vi "Configure Trigger (USB).vi"(0 "VISA resource name":refnum<visa-resource-name>, 1 "Split Transaction Start/End (0: No Care)":u16(ring) items=["No Care", "Full Speed", "Low Speed", "ISO Start", "ISO Middle", "ISO End", "ISO All"], 2 "Split Transaction Field (0: No Care)":u16(ring) items=["No Care", "S Split", "C Split"], 5 "Trigger Source (9: Bus 1)":u16(ring)=9 items=["Bus 1"=9, "Bus 2"=10], 7 "Split Transaction Hub Address (\"XXXXXXX\")":string="XXXXXXX", 9 "Split Transaction Port Address (\"XXXXXXX\")":string="XXXXXXX", 11 "error in (no error)":errorcluster, 12 "Split Transaction Endpoint (0: No Care)":u16(ring) items=["No Care", "Control", "ISO", "Bulk", "Interrupt"]) -> (4 "VISA resource name out":refnum<visa-resource-name>, 15 "error out":errorcluster)   [LabVIEW 2013, in "Tektronix DPO MSO 2000 4000 Series.lvlib"]
doc: "Configures USB trigger settings for an oscilloscope. \n\n<B>Note:</B>\nThis VI only applies to DPO4034B, DPO4054B, DPO4104B, MSO4034B, MSO4054B, MSO4104B."
uses:
  Tektronix DPO MSO 2000 4000 Series.lvlib
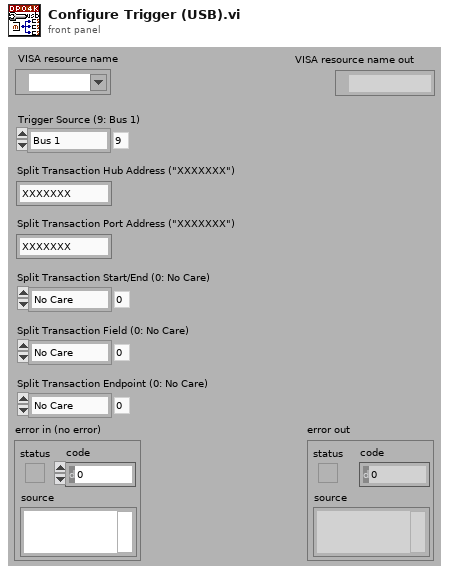
[diagram p1: front panel]
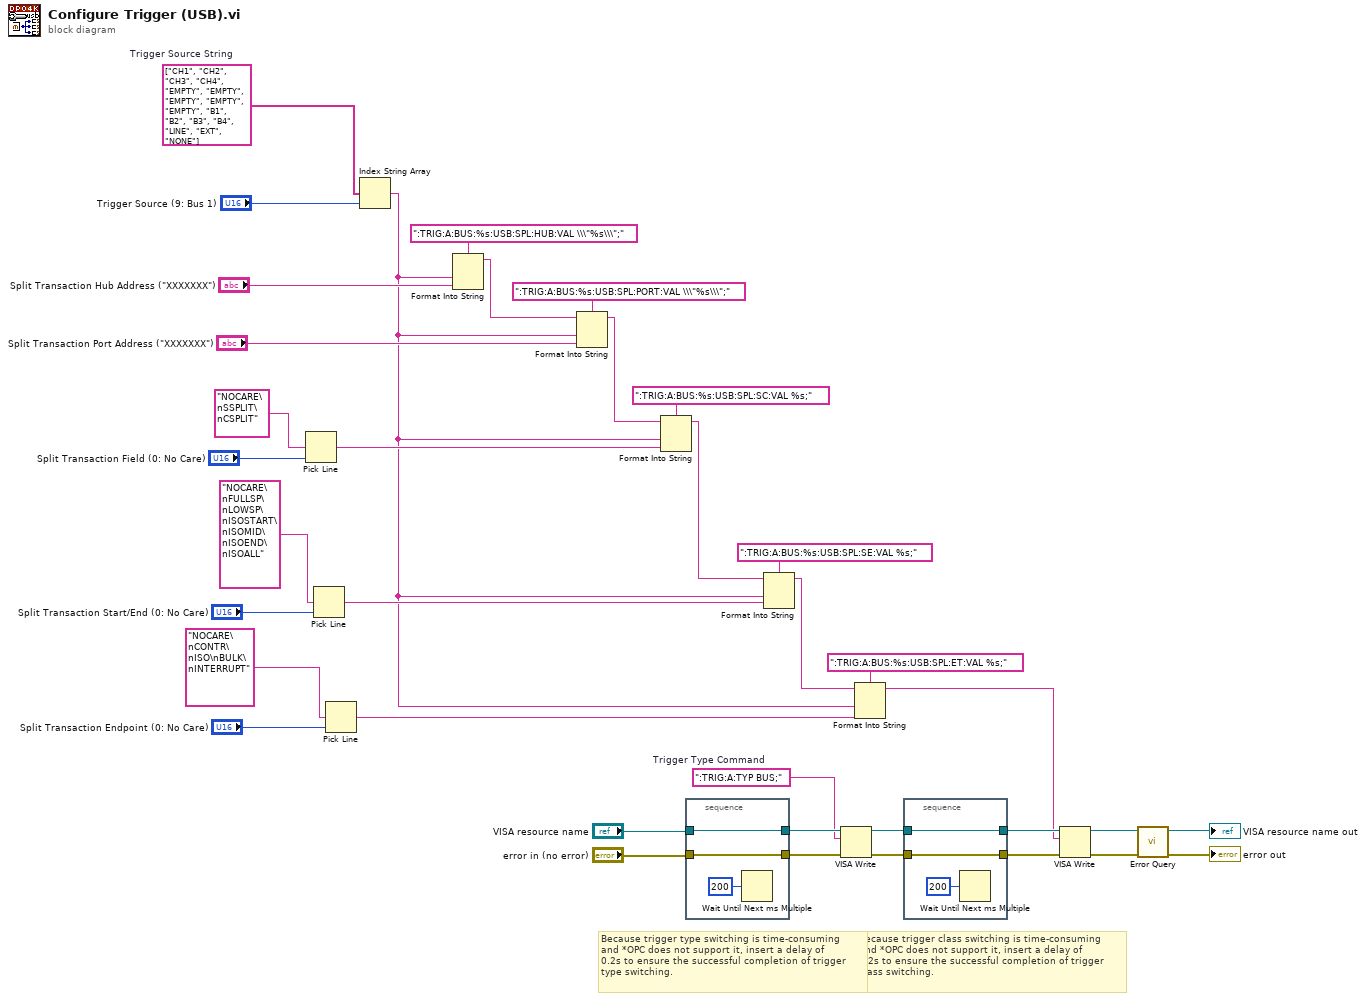
[diagram p0: block diagram]
diagram:
  w30 = string[] ["CH1", "CH2", "CH3", "CH4", "EMPTY", "EMPTY", "EMPTY", "EMPTY", "EMPTY", "B1", "B2", "B3", "B4", "LINE", "EXT", "NONE"]  # Trigger Source String
  w35 = ":TRIG:A:TYP BUS;"  # Trigger Type Command
  # "Because trigger class switching is time-consuming\nand *OPC does not support it, insert a delay of\n0.2s to ensure the successful completion of trigger\nclass switching."
  # "Because trigger type switching is time-consuming\nand *OPC does not support it, insert a delay of\n0.2s to ensure the successful completion of trigger\ntype switching."
  n1 = Pick Line(multi-line string="NOCARE\nSSPLIT\nCSPLIT", line index="Split Transaction Field (0: No Care)") -> (output string=w15:string)  [unwired: 1 in]
  n2 = Pick Line(multi-line string="NOCARE\nFULLSP\nLOWSP\nISOSTART\nISOMID\nISOEND\nISOALL", line index="Split Transaction Start/End (0: No Care)") -> (output string=w10:string)  [unwired: 1 in]
  n3 = Pick Line(multi-line string="NOCARE\nCONTR\nISO\nBULK\nINTERRUPT", line index="Split Transaction Endpoint (0: No Care)") -> (output string=w4:string)  [unwired: 1 in]
  n4 = Index String Array(1:"Trigger Source (9: Bus 1)", 2:w30) -> (0:w5:string)  [unwired: 1 in]
  n5 = Format Into String(format string=":TRIG:A:BUS:%s:USB:SPL:HUB:VAL \\\"%s\\\";", w5, "Split Transaction Hub Address (\"XXXXXXX\")") -> (resulting string=w2:string)  [unwired: 2 in, 1 out]
  n6 = Format Into String(format string=":TRIG:A:BUS:%s:USB:SPL:PORT:VAL \\\"%s\\\";", initial string=w2, w5, "Split Transaction Port Address (\"XXXXXXX\")") -> (resulting string=w3:string)  [unwired: 1 in, 1 out]
  n7 = Format Into String(format string=":TRIG:A:BUS:%s:USB:SPL:SC:VAL %s;", initial string=w3, w5, w15) -> (resulting string=w12:string)  [unwired: 1 in, 1 out]
  n8 = stacked-sequence {
    tunnel: "VISA resource name" -> [w39]
    tunnel: [w39] -> w37
    tunnel: "error in (no error)" -> [w38]
    tunnel: [w38] -> w36
    frame #0 {
      n9 = Wait Until Next ms Multiple(millisecond multiple=u32 200) -> ()  [unwired: 1 out]
    }
  }
  n10 = Format Into String(format string=":TRIG:A:BUS:%s:USB:SPL:SE:VAL %s;", initial string=w12, w5, w10) -> (resulting string=w6:string)  [unwired: 1 in, 1 out]
  n11 = VISA Write(VISA resource name=w37, write buffer=w35, error in (no error)=w36) -> (VISA resource name out=w34:refnum<visa-resource-name>, error out=w33:errorcluster)  [unwired: 1 out]
  n12 = Format Into String(format string=":TRIG:A:BUS:%s:USB:SPL:ET:VAL %s;", initial string=w6, w5, w4) -> (resulting string=w1:string)  [unwired: 1 in, 1 out]
  n13 = stacked-sequence {
    tunnel: w34 -> [w42]
    tunnel: [w42] -> w32
    tunnel: w33 -> [w41]
    tunnel: [w41] -> w31
    frame #0 {
      n14 = Wait Until Next ms Multiple(millisecond multiple=u32 200) -> ()  [unwired: 1 out]
    }
  }
  n15 = VISA Write(VISA resource name=w32, write buffer=w1, error in (no error)=w31) -> (VISA resource name out=w28:refnum<visa-resource-name>, error out=w27:errorcluster)  [unwired: 1 out]
  n16 = call "Error Query.vi"("error in (no error)"=w27, "VISA resource name"=w28) -> ("error out"=→"error out":errorcluster, "VISA resource name out"=→"VISA resource name out":refnum<visa-resource-name>)  [unwired: 6 in, 2 out]
